vi "Trim Input JSON (and make Object).vi"(11 "JSON Input":string) -> (3 "<JSON>Object":string)   [LabVIEW 2015, in "JSONtext.lvlib"]
uses:
  JSONtext.lvlib
panel:
  # "Make empty input count as null"
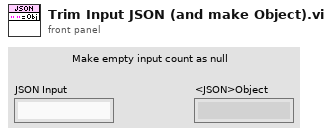
[diagram p1: front panel]
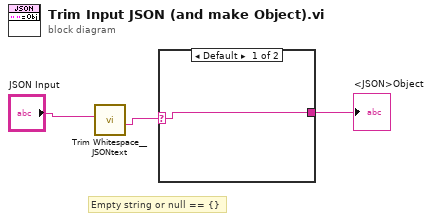
[diagram p0: block diagram]
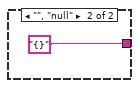
[diagram p2: hidden frame]
diagram:
  # "Empty string or null == {}"
  n1 = call "Trim Whitespace__JSONtext.vi"("String in"="JSON Input") -> ("String out"=w2:string)  [unwired: 6 in]
  n2 = case shown="Default" w2 {
    selector: w2 -> [w4 _]
    tunnel: [w4 "{}"] -> w1
    frame Default {
    }
    frame "", "null" {
    }
  }
  "<JSON>Object" <- w1
